vi "removeObserver.vi"(8 "error in (no error)":errorcluster, 10 "Observer.lvclass":refnum<class "Observer.lvclass">, 11 "WeatherData.lvclass":refnum<class "WeatherData.lvclass">) -> (0 "error out":errorcluster, 3 "WeatherData.lvclass 2":refnum<class "WeatherData.lvclass">)   [LabVIEW 2020, in "WeatherData.lvclass"]
uses:
  WeatherData.lvclass
  Observer/Observer.lvclass
  WeatherData.lvclass/WeatherData.ctl
panel:
  # "Connector Pane"
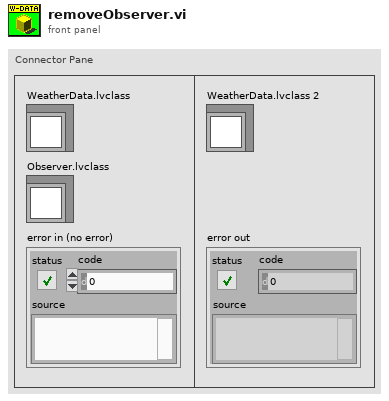
[diagram p1: front panel]
types:
  T1 = typedef "weatherDataCluster.ctl" = cluster{"Temperature":dbl, "Humidity":dbl, "Pressure":dbl, "Observers":refnum<class "Observer.lvclass">[]}
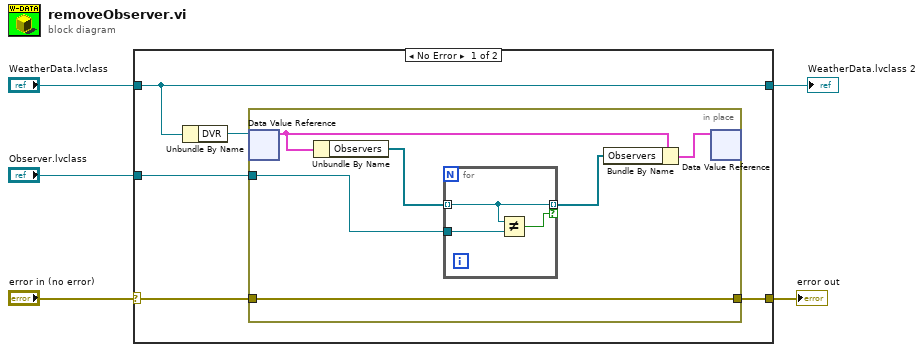
[diagram p0: block diagram]
diagram:
  n1 = case shown="No Error" "error in (no error)" {
    selector: "error in (no error)" -> [w8 w20]
    tunnel: "Observer.lvclass" -> [w10 _]
    tunnel: [w9 w20] -> w4
    tunnel: "WeatherData.lvclass" -> [w6 w21]
    tunnel: [w6 w21] -> w1
    frame No Error {
      n2 = Unbundle By Name(w6) -> ("DVR"=w7:refnum<data-value>)
      n3 = in-place {
        in-place-border: w10 -> [w16]
        in-place-border: [w15] -> w9
        in-place-border: w8 -> [w15]
        n4 = in-place-dvr #1(w7) -> (w13:T1)  [unwired: 1 out]
        n5 = Unbundle By Name(w13) -> ("Observers"=w14:refnum<class "Observer.lvclass">[])
        n6 = for {
          tunnel: w14 -> [w18] mode=indexing
          tunnel: w16 -> [w19]
          tunnel: [w18] -> w11 mode=indexing if=w17
          n7 = Not Equal?(x=w18, y=w19) -> (x != y?=w17:bool)
        }
        n8 = Bundle By Name(cluster=w13, "Observers"=w11) -> (w12:T1)
        n9 = in-place-dvr #1(w12) -> ()  [unwired: 2 out]
      }
    }
    frame Error {
    }
  }
  "error out" <- w4
  "WeatherData.lvclass 2" <- w1
